vi "CANdleGetters.vi"   [LabVIEW 2025]
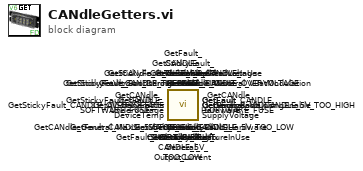
[diagram p0: block diagram]
diagram:
  n1 = call <vilib>:"GetStickyFault_CANDLE_SHORT_CIRCUIT.vi"() -> ()  [unwired: 10 in, 2 out]
  n2 = call <vilib>:"GetFault_CANDLE_SHORT_CIRCUIT.vi"() -> ()  [unwired: 10 in, 2 out]
  n3 = call <vilib>:"GetStickyFault_CANDLE_SOFTWARE_FUSE.vi"() -> ()  [unwired: 10 in, 2 out]
  n4 = call <vilib>:"GetFault_CANDLE_SOFTWARE_FUSE.vi"() -> ()  [unwired: 10 in, 2 out]
  n5 = call <vilib>:"GetStickyFault_CANDLE_THERMAL.vi"() -> ()  [unwired: 10 in, 2 out]
  n6 = call <vilib>:"GetFault_CANDLE_THERMAL.vi"() -> ()  [unwired: 10 in, 2 out]
  n7 = call <vilib>:"GetStickyFault_CANDLE_5V_TOO_LOW.vi"() -> ()  [unwired: 10 in, 2 out]
  n8 = call <vilib>:"GetFault_CANDLE_5V_TOO_LOW.vi"() -> ()  [unwired: 10 in, 2 out]
  n9 = call <vilib>:"GetStickyFault_CANDLE_5V_TOO_HIGH.vi"() -> ()  [unwired: 10 in, 2 out]
  n10 = call <vilib>:"GetFault_CANDLE_5V_TOO_HIGH.vi"() -> ()  [unwired: 10 in, 2 out]
  n11 = call <vilib>:"GetStickyFault_CANDLE_OVERVOLTAGE.vi"() -> ()  [unwired: 10 in, 2 out]
  n12 = call <vilib>:"GetFault_CANDLE_OVERVOLTAGE.vi"() -> ()  [unwired: 10 in, 2 out]
  n13 = call <vilib>:"GetStickyFault_UnlicensedFeatureInUse.vi"() -> ()  [unwired: 10 in, 2 out]
  n14 = call <vilib>:"GetFault_UnlicensedFeatureInUse.vi"() -> ()  [unwired: 10 in, 2 out]
  n15 = call <vilib>:"GetStickyFault_BootDuringEnable.vi"() -> ()  [unwired: 10 in, 2 out]
  n16 = call <vilib>:"GetFault_BootDuringEnable.vi"() -> ()  [unwired: 10 in, 2 out]
  n17 = call <vilib>:"GetStickyFault_Undervoltage.vi"() -> ()  [unwired: 10 in, 2 out]
  n18 = call <vilib>:"GetFault_Undervoltage.vi"() -> ()  [unwired: 10 in, 2 out]
  n19 = call <vilib>:"GetStickyFault_Hardware.vi"() -> ()  [unwired: 10 in, 2 out]
  n20 = call <vilib>:"GetFault_Hardware.vi"() -> ()  [unwired: 10 in, 2 out]
  n21 = call <vilib>:"GetCANdle_General_MaxSimulAnimCount.vi"() -> ()  [unwired: 10 in, 2 out]
  n22 = call <vilib>:"GetCANdle_General_VBatModulation.vi"() -> ()  [unwired: 10 in, 2 out]
  n23 = call <vilib>:"GetCANdle_General_DeviceTemp.vi"() -> ()  [unwired: 10 in, 2 out]
  n24 = call <vilib>:"GetCANdle_General_OutputCurrent.vi"() -> ()  [unwired: 10 in, 2 out]
  n25 = call <vilib>:"GetCANdle_General_FiveVRailVoltage.vi"() -> ()  [unwired: 10 in, 2 out]
  n26 = call <vilib>:"GetCANdle_General_SupplyVoltage.vi"() -> ()  [unwired: 10 in, 2 out]
  n27 = call <vilib>:"GetVersion_IsProLicensed.vi"() -> ()  [unwired: 10 in, 2 out]
  n28 = call <vilib>:"GetAllStickyFaults.vi"() -> ()  [unwired: 10 in, 2 out]
  n29 = call <vilib>:"GetAllFaults.vi"() -> ()  [unwired: 10 in, 2 out]
  n30 = call <vilib>:"GetVersion_Full.vi"() -> ()  [unwired: 10 in, 2 out]
  n31 = call <vilib>:"GetVersion_Build.vi"() -> ()  [unwired: 10 in, 2 out]
  n32 = call <vilib>:"GetVersion_Bugfix.vi"() -> ()  [unwired: 10 in, 2 out]
  n33 = call <vilib>:"GetVersion_Minor.vi"() -> ()  [unwired: 10 in, 2 out]
  n34 = call <vilib>:"GetVersion_Major.vi"() -> ()  [unwired: 10 in, 2 out]
